vi "Cryo-Con -- Identify.vi"(8 "Error In":errorcluster, 11 "VISA resource name":refnum<visa-resource-name>) -> (0 "Error Out":errorcluster, 1 "data string out":string, 2 "Cryo-con":bool, 3 "VISA resource name out":refnum<visa-resource-name>)   [LabVIEW 2017]
uses:
  NHMFL_Core/Libraries/Instruments/GPIB/VISA  Send Receive.vi
panel:
  in  "Serial Configuration":cluster{"Baud Rate":u32}={"Baud Rate"=9600} {"Baud Rate" items=["300"=300, "600"=600, "1200"=1200, "2400"=2400, "4800"=4800, "9600"=9600, "19200"=19200]}
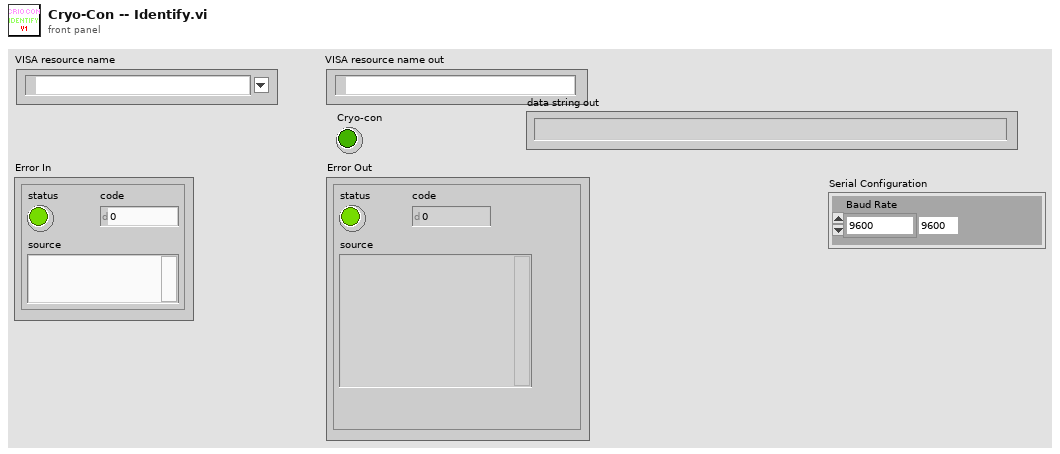
[diagram p1: front panel]
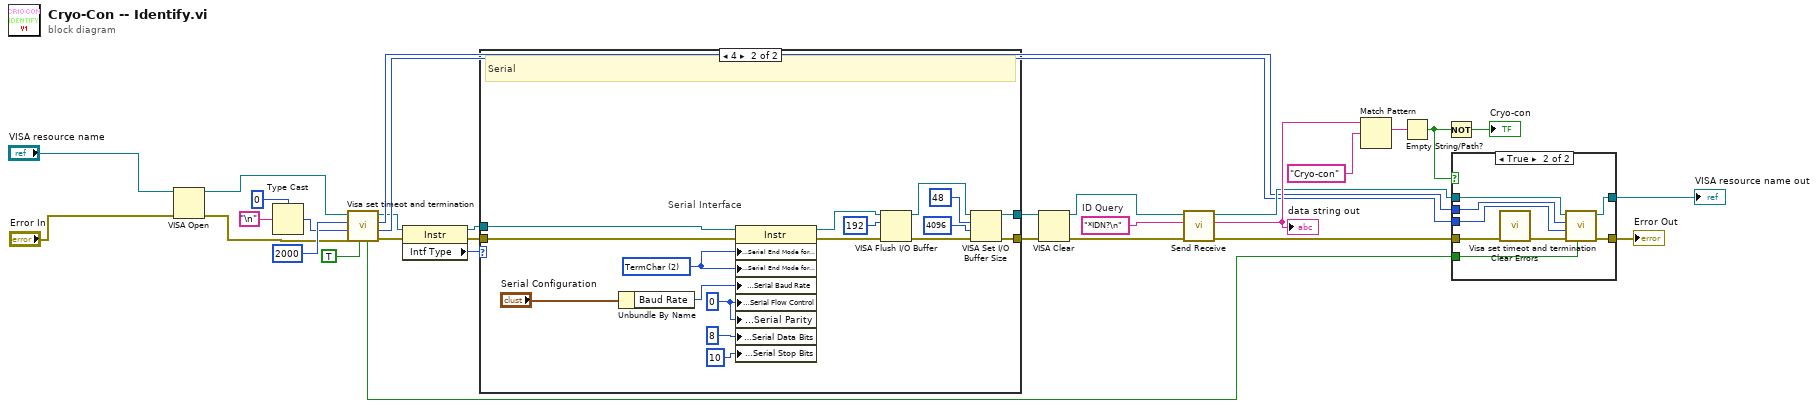
[diagram p0: block diagram]
diagram:
  w29 = "*IDN?\n"  # ID Query
  n1 = VISA Open(error in (no error)="Error In", VISA resource name="VISA resource name") -> (VISA resource name=w3:refnum<visa-resource-name>, error out=w1:errorcluster)  [unwired: 3 in]
  n2 = Type Cast(type=u8 0, x="\n" ("Line Feed Constant")) -> (*(type *) &x=w12:u8)
  n3 = call "Visa set timeot and termination.vi"("Termination Character Enable"=TRUE ("Message Based Settings:Termination Character Enable"), "error in (no error)"=w1, "Termination Character"=w12, "Timeout Value"=u32 2000 ("General Settings:Timeout Value"), "VISA resource name"=w3) -> ("error out"=w15:errorcluster, "Old Termination Character"=w10:u8, "Old Timeout Value"=w11:u32, "VISA resource name out"=w7:refnum<visa-resource-name>, "Old Termination Character Enable"=w9:bool)  [unwired: 2 in]
  n4 = property class="Instr"(reference=w7, error in=w15) -> (reference out=w6:refnum<visa-resource-name>, error out=w8:errorcluster, "Intf Type"=w5:u16)
  n5 = case shown="4" w5 {
    tunnel: [w32 w47] -> w17
    tunnel: [w33 w44] -> w16
    tunnel: w6 -> [w32 w49]
    tunnel: w8 -> [w33 w50]
    frame 0, Default {
      # "TCP/IP uses end-of-line char of \\n to terminate reads"
      # "GPIB and TCP/IP Interfaces"
    }
    frame 4 {
      w36 = u16 0
      w39 = u16 2 items=["None", "LastBit", "TermChar"] ("Serial Settings:Serial End Mode for Reads")
      # "Serial Interface"
      # "Serial"
      n6 = Unbundle By Name("Serial Configuration") -> ("Baud Rate"=w38:u32)
      n7 = property class="Instr"(reference=w49, error in=w50, "Serial Settings:Serial End Mode for Reads"=w39, "Serial Settings:Serial End Mode for Writes"=w39, "Serial Settings:Serial Baud Rate"=w38, "Serial Settings:Serial Flow Control"=w36, "Serial Settings:Serial Parity"=w36, "Serial Settings:Serial Data Bits"=u16 8, "Serial Settings:Serial Stop Bits"=u16 10) -> (reference out=w43:refnum<visa-resource-name>, error out=w46:errorcluster)
      n8 = VISA Flush I/O Buffer(VISA resource name=w43, mask (16)=u16 192, error in (no error)=w46) -> (VISA resource name out=w48:refnum<visa-resource-name>, error out=w45:errorcluster)
      n9 = VISA Set I/O Buffer Size(VISA resource name=w48, mask (16)=u16 48, size (4096)=u32 4096 ("size (0)"), error in (no error)=w45) -> (VISA resource name out=w47:refnum<visa-resource-name>, error out=w44:errorcluster)
    }
  }
  n10 = VISA Clear(VISA resource name=w17, error in (no error)=w16) -> (VISA resource name out=w19:refnum<visa-resource-name>, error out=w18:errorcluster)
  n11 = call-poly "Send Receive.vi"("error in (no error)"=w18, "data string in"=w29, "VISA Resource Name"=w19) -> ("error out"=w23:errorcluster, "data string out"=w28:string, "VISA Resource Name Out"=w22:refnum<visa-resource-name>)  [unwired: 6 in]
  "data string out" <- w28
  n12 = Match Pattern(string=w28, regular expression="Cryo-con") -> (match substring=w26:string)  [unwired: 1 in, 3 out]
  n13 = Empty String/Path?(string/path=w26) -> (empty?=w24:bool)
  n14 = Not(x=w24) -> (.not. x?=→"Cryo-con":bool)
  n15 = case shown="True" w24 {
    tunnel: w23 -> [w52 w60]
    tunnel: w22 -> [w51 w59]
    tunnel: w11 -> [_ w57]
    tunnel: w9 -> [_ w56]
    tunnel: w10 -> [_ w55]
    tunnel: [w52 w53] -> w21
    tunnel: [w51 w58] -> w20
    frame False {
    }
    frame True {
      n16 = call <vilib>:"Clear Errors.vi"("error in (no error)"=w60) -> ("error out"=w54:errorcluster)  [unwired: 5 in, 1 out]
      n17 = call "Visa set timeot and termination.vi"("Termination Character Enable"=w56, "error in (no error)"=w54, "Termination Character"=w55, "Timeout Value"=w57, "VISA resource name"=w59) -> ("error out"=w53:errorcluster, "VISA resource name out"=w58:refnum<visa-resource-name>)  [unwired: 2 in, 3 out]
    }
  }
  "VISA resource name out" <- w20
  "Error Out" <- w21
